vi "get preset name.vi"(1 "Cluster in":T1={"Country 1 index"=201, "Country 2 index"=0, "countries"=[], "Data"=0, "Curve fit all data"=TRUE, "Curve 1 type"=enum."Exponential", "Curve 2 type"=enum."Exponential", "absolute?"=TRUE, "cursor 1 "=0.0, "cursor 2 "=0.0, "threshold cases"=1} {"Data" items=["cumulative cases", "new cases per day", "deaths"]}) -> (0 "Preset name out":string)   [LabVIEW 2019]
panel:
  in  "OK Button":bool
  in  "Preset name":string
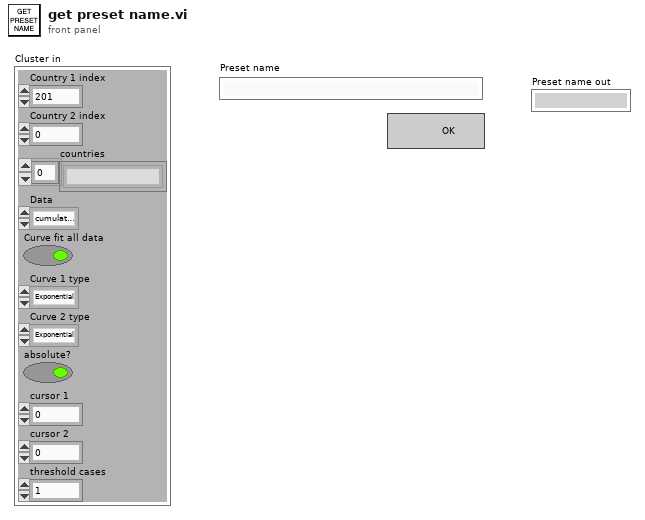
[diagram p1: front panel]
types:
  T1 = cluster{"Country 1 index":i32, "Country 2 index":i32, "countries":string[], "Data":u16, "Curve fit all data":bool, "Curve 1 type":enum16{"Exponential", "Logarithm"}, "Curve 2 type":enum16{"Exponential", "Logarithm"}, "absolute?":bool, "cursor 1 ":dbl, "cursor 2 ":dbl, "threshold cases":u32}
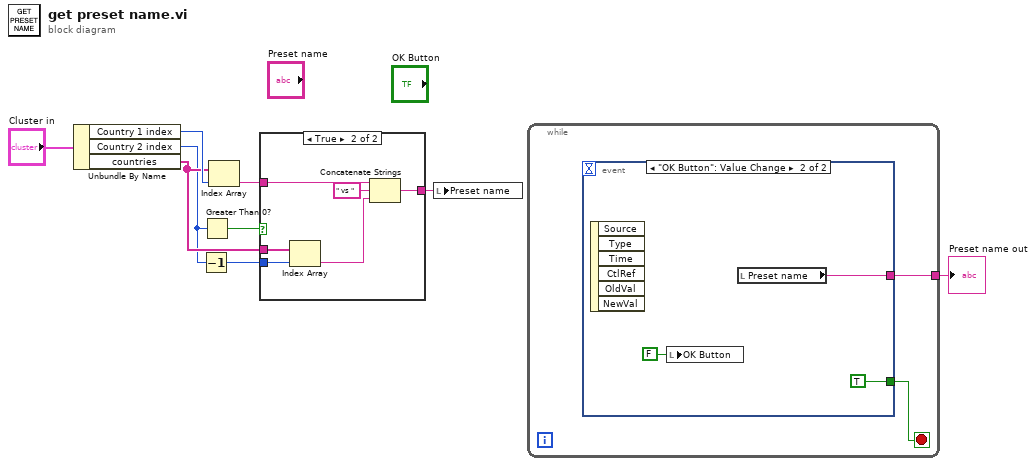
[diagram p0: block diagram]
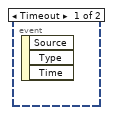
[diagram p3: hidden frame]
diagram:
  n1 = Unbundle By Name("Cluster in") -> ("Country 1 index"=w8:i32, "Country 2 index"=w4:i32, "countries"=w5:string[])
  n2 = Decrement(x=w4) -> (x-1=w2:i32)
  n3 = Greater Than 0?(x=w4) -> (x > 0?=w7:bool)
  n4 = Index Array(array=w5, index=w8) -> (element=w6:string)
  n5 = case shown="True" w7 {
    tunnel: w6 -> [w10 w16]
    tunnel: w5 -> [_ w14]
    tunnel: w2 -> [_ w13]
    tunnel: [w10 w11] -> w3
    frame False {
    }
    frame True {
      n6 = Index Array(array=w14, index=w13) -> (element=w12:string)
      n7 = Concatenate Strings(w16, " vs " ("string"), w12) -> (w11:string)
    }
  }
  n8 = local write "Preset name"(w3) -> ()
  n9 = while {
    tunnel: [w18] -> w9
    stop <- w17 stop-if-true
    n10 = event shown="[1] \"OK Button\": Value Change" {
      selector: _ -> [_ _]
      dyn-events: _ -> [_ _]
      timeout: _ -> [_ _]
      tunnel: [_ w20] -> w18
      tunnel: [_ TRUE] -> w17
      event Timeout {
        n11 = event-data() -> ()  [unwired: 1 in, 3 out]
      }
      event "OK Button": Value Change {
        n12 = event-data() -> ()  [unwired: 1 in, 6 out]
        n13 = local write "OK Button"(FALSE ("OK Button")) -> ()
        n14 = local read "Preset name"() -> (w20:string)
      }
    }
  }
  "Preset name out" <- w9
